vi "test_read-nmea-data2.vi"() -> ()   [LabVIEW 2019] (continued)
\t\n15:13:37.95\tF9P\t\t\n15:13:37.97\tF9P\t\t\n15:13:37.99\tF9P\t\t\n15:13:38.01\tF9P\t\t\n15:13:38.03\tF9P\t\t\n15:13:38.05\tF9P\t\t\n15:13:38.07\tF9P\t\t\n15:13:38.09\tF9P\t\t\n15:13:38.11\tF9P\t\t\n15:13:38.13\tF9P\t\t\n15:13:38.15\tF9P\t\t\n15:13:38.17\tF9P\t\t\n15:13:38.19\tF9P\t\t\n15:13:38.21\tF9P\t\t\n15:13:38.23\tF9P\t$GNRMC,061340.00,A,3723.56861,N,12656.98776,E,1.974,335.21,250720,,,A,V*0D\n\t\n15:13:38.25\tF9P\t$GNVTG,335.21,T,,M,1.974,N,3.655,K,A*2B\n\t\n15:13:38.27\tF9P\t$GNGGA,061340.00,3723.56861,N,12656.98776,E,1,12,1.09,47.7,M,18.5,M,,*79\n\t\n15:13:38.29\tF9P\t$GNGSA,A,3,12,06,19,05,17,09,04,02,,,,,2.14,1.09,1.84,1*02\n\t\n15:13:38.31\tF9P\t$GNGSA,A,3,85,70,71,84,,,,,,,,,2.14,1.09,1.84,2*00\n\t\n15:13:38.33\tF9P\t$GNGSA,A,3,36,19,11,04,09,12,,,,,,,2.14,1.09,1.84,3*02\n\t\n15:13:38.35\tF9P\t$GNGSA,A,3,14,11,33,,,,,,,,,,2.14,1.09,1.84,4*03\n\t\n15:13:38.37\tF9P\t$GPGSV,3,1,09,02,55,320,29,04,17,043,18,05,38,248,26,06,64,050,38,1*65\n\t\n15:13:38.39\tF9P\t$GPGSV,3,2,09,09,44,073,30,12,23,276,33,17,32,154,33,19,51,157,37,1*6F\n\t\n15:13:38.41\tF9P\t$GPGSV,3,3,09,25,12,306,23,1*5D\n\t\n15:13:38.43\tF9P\t$GPGSV,3,1,09,02,55,320,,04,17,043,,05,38,248,,06,64,050,25,6*68\n\t\n15:13:38.45\tF9P\t$GPGSV,3,2,09,09,44,073,27,12,23,276,30,17,32,154,23,19,51,157,,6*68\n\t\n15:13:38.47\tF9P\t$GPGSV,3,3,09,25,12,306,,6*5B\n\t\n15:13:38.49\tF9P\t$GLGSV,2,1,08,69,11,031,33,70,70,038,25,71,53,206,30,72,05,210,17,1*70\n\t\n15:13:38.51\tF9P\t$GLGSV,2,2,08,77,01,325,,84,19,123,17,85,70,070,33,86,37,330,,1*70\n\t\n15:13:38.53\tF9P\t$GLGSV,2,1,08,69,11,031,20,70,70,038,,71,53,206,23,72,05,210,,3*73\n\t\n15:13:38.55\tF9P\t$GLGSV,2,2,08,77,01,325,,84,19,123,20,85,70,070,22,86,37,330,,3*76\n\t\n15:13:38.57\tF9P\t$GAGSV,2,1,08,02,08,297,11,04,66,116,31,09,32,193,35,11,72,359,24,7*77\n\t\n15:13:38.59\tF9P\t$GAGSV,2,2,08,12,40,103,29,19,26,045,16,25,09,249,,36,26,308,14,7*71\n\t\n15:13:38.61\tF9P\t$GAGSV,2,1,08,02,08,297,,04,66,116,,09,32,193,,11,72,359,,2*70\n\t\n15:13:38.63\tF9P\t$GAGSV,2,2,08,12,40,103,,19,26,045,,25,09,249,,36,26,308,,2*7D\n\t\n15:13:38.65\tF9P\t$GBGSV,1,1,04,11,49,132,30,14,87,114,27,28,,,34,33,61,220,21,1*4E\n\t\n15:13:38.67\tF9P\t$GBGSV,1,1,03,11,49,132,34,14,87,114,,33,61,220,,3*44\n\t\n15:13:38.69\tF9P\t$GNGLL,3723.56861,N,12656.98776,E,061340.00,A,A*7F\n\t\n15:13:38.71\tF9P\t\t\n15:13:38.73\tF9P\t\t\n15:13:38.75\tF9P\t\t\n15:13:38.77\tF9P\t\t\n15:13:38.79\tF9P\t\t\n15:13:38.81\tF9P\t\t\n15:13:38.83\tF9P\t\t\n15:13:38.85\tF9P\t\t\n15:13:38.87\tF9P\t\t\n15:13:38.89\tF9P\t\t\n15:13:38.91\tF9P\t\t\n15:13:38.93\tF9P\t\t\n15:13:38.95\tF9P\t\t\n15:13:38.97\tF9P\t\t\n15:13:38.99\tF9P\t\t\n15:13:39.01\tF9P\t\t\n15:13:39.03\tF9P\t\t\n15:13:39.05\tF9P\t\t\n15:13:39.07\tF9P\t\t\n15:13:39.09\tF9P\t\t\n15:13:39.11\tF9P\t\t\n15:13:39.13\tF9P\t\t\n15:13:39.15\tF9P\t\t\n15:13:39.17\tF9P\t\t\n15:13:39.19\tF9P\t\t\n15:13:39.21\tF9P\t\t\n15:13:39.23\tF9P\t$GNRMC,061341.00,A,3723.56927,N,12656.98763,E,2.191,340.11,250720,,,A,V*0A\n\t\n15:13:39.25\tF9P\t$GNVTG,340.11,T,,M,2.191,N,4.057,K,A*29\n\t\n15:13:39.27\tF9P\t$GNGGA,061341.00,3723.56927,N,12656.98763,E,1,12,1.09,47.1,M,18.5,M,,*79\n\t\n15:13:39.29\tF9P\t$GNGSA,A,3,12,06,19,05,17,09,04,02,,,,,2.14,1.09,1.84,1*02\n\t\n15:13:39.31\tF9P\t$GNGSA,A,3,85,70,71,84,,,,,,,,,2.14,1.09,1.84,2*00\n\t\n15:13:39.33\tF9P\t$GNGSA,A,3,36,19,11,04,09,12,,,,,,,2.14,1.09,1.84,3*02\n\t\n15:13:39.35\tF9P\t$GNGSA,A,3,14,11,33,,,,,,,,,,2.14,1.09,1.84,4*03\n\t\n15:13:39.37\tF9P\t$GPGSV,3,1,09,02,55,320,32,04,17,043,19,05,38,248,25,06,64,050,31,1*64\n\t\n15:13:39.39\tF9P\t$GPGSV,3,2,09,09,44,073,36,12,23,276,37,17,32,154,36,19,51,157,41,1*69\n\t\n15:13:39.41\tF9P\t$GPGSV,3,3,09,25,12,306,23,1*5D\n\t\n15:13:39.43\tF9P\t$GPGSV,3,1,09,02,55,320,,04,17,043,,05,38,248,,06,64,050,25,6*68\n\t\n15:13:39.45\tF9P\t$GPGSV,3,2,09,09,44,073,28,12,23,276,28,17,32,154,24,19,51,157,,6*69\n\t\n15:13:39.47\tF9P\t$GPGSV,3,3,09,25,12,306,,6*5B\n\t\n15:13:39.49\tF9P\t$GLGSV,2,1,08,69,11,031,19,70,70,038,24,71,53,206,29,72,05,210,17,1*71\n\t\n15:13:39.51\tF9P\t$GLGSV,2,2,08,77,01,325,,84,19,123,17,85,70,070,29,86,37,330,,1*7B\n\t\n15:13:39.53\tF9P\t$GLGSV,2,1,08,69,11,031,20,70,70,038,,71,53,206,22,72,05,210,,3*72\n\t\n15:13:39.55\tF9P\t$GLGSV,2,2,08,77,01,325,,84,19,123,21,85,70,070,21,86,37,330,,3*74\n\t\n15:13:39.57\tF9P\t$GAGSV,2,1,08,02,08,297,09,04,66,116,26,09,32,193,28,11,72,359,25,7*75\n\t\n15:13:39.59\tF9P\t$GAGSV,2,2,08,12,40,103,30,19,26,045,16,25,09,249,,36,26,308,14,7*79\n\t\n15:13:39.61\tF9P\t$GAGSV,2,1,08,02,08,297,,04,66,116,,09,32,193,,11,72,359,,2*70\n\t\n15:13:39.63\tF9P\t$GAGSV,2,2,08,12,40,103,,19,26,045,,25,09,249,,36,26,308,,2*7D\n\t\n15:13:39.65\tF9P\t$GBGSV,1,1,04,11,49,132,31,14,87,114,32,28,,,25,33,61,220,21,1*4B\n\t\n15:13:39.67\tF9P\t$GBGSV,1,1,03,11,49,132,31,14,87,114,31,33,61,220,,3*43\n\t\n15:13:39.69\tF9P\t$GNGLL,3723.56927,N,12656.98763,E,061341.00,A,A*79\n\t\n15:13:39.71\tF9P\t\t\n15:13:39.73\tF9P\t\t\n15:13:39.75\tF9P\t\t\n15:13:39.77\tF9P\t\t\n15:13:39.79\tF9P\t\t\n15:13:39.81\tF9P\t\t\n15:13:39.83\tF9P\t\t\n15:13:39.85\tF9P\t\t\n15:13:39.87\tF9P\t\t\n15:13:39.89\tF9P\t\t\n15:13:39.91\tF9P\t\t\n15:13:39.93\tF9P\t\t\n15:13:39.95\tF9P\t\t\n15:13:39.97\tF9P\t\t\n15:13:39.99\tF9P\t\t\n15:13:40.01\tF9P\t\t\n15:13:40.03\tF9P\t\t\n15:13:40.05\tF9P\t\t\n15:13:40.07\tF9P\t\t\n15:13:40.09\tF9P\t\t\n15:13:40.11\tF9P\t\t\n15:13:40.13\tF9P\t\t\n15:13:40.15\tF9P\t\t\n15:13:40.17\tF9P\t\t\n15:13:40.19\tF9P\t\t\n15:13:40.21\tF9P\t\t\n15:13:40.23\tF9P\t$GNRMC,061342.00,A,3723.56991,N,12656.98768,E,1.862,343.66,250720,,,A,V*0A\n\t\n15:13:40.25\tF9P\t$GNVTG,343.66,T,,M,1.862,N,3.449,K,A*20\n\t\n15:13:40.27\tF9P\t$GNGGA,061342.00,3723.56991,N,12656.98768,E,1,12,1.09,46.8,M,18.5,M,,*74\n\t\n15:13:40.29\tF9P\t$GNGSA,A,3,12,06,19,05,17,09,04,02,,,,,2.14,1.09,1.84,1*02\n\t\n15:13:40.31\tF9P\t$GNGSA,A,3,85,70,71,84,,,,,,,,,2.14,1.09,1.84,2*00\n\t\n15:13:40.33\tF9P\t$GNGSA,A,3,36,19,11,04,09,12,,,,,,,2.14,1.09,1.84,3*02\n\t\n15:13:40.35\tF9P\t$GNGSA,A,3,14,11,33,,,,,,,,,,2.14,1.09,1.84,4*03\n\t\n15:13:40.37\tF9P\t$GPGSV,3,1,09,02,55,320,27,04,17,043,20,05,38,248,26,06,64,050,35,1*6D\n\t\n15:13:40.39\tF9P\t$GPGSV,3,2,09,09,44,073,38,12,23,276,32,17,32,154,31,19,51,157,37,1*64\n\t\n15:13:40.41\tF9P\t$GPGSV,3,3,09,25,12,306,20,1*5E\n\t\n15:13:40.43\tF9P\t$GPGSV,3,1,09,02,55,320,,04,17,043,,05,38,248,,06,64,050,26,6*6B\n\t\n15:13:40.45\tF9P\t$GPGSV,3,2,09,09,44,073,28,12,23,276,21,17,32,154,25,19,51,157,,6*61\n\t\n15:13:40.47\tF9P\t$GPGSV,3,3,09,25,12,306,,6*5B\n\t\n15:13:40.49\tF9P\t$GLGSV,2,1,08,69,11,031,29,70,70,038,25,71,53,206,29,72,05,210,17,1*73\n\t\n15:13:40.51\tF9P\t$GLGSV,2,2,08,77,01,325,,84,19,123,19,85,70,070,32,86,37,330,,1*7F\n\t\n15:13:40.53\tF9P\t$GLGSV,2,1,08,69,11,031,20,70,70,038,,71,53,206,20,72,05,210,,3*70\n\t\n15:13:40.55\tF9P\t$GLGSV,2,2,08,77,01,325,,84,19,123,24,85,70,070,21,86,37,330,,3*71\n\t\n15:13:40.57\tF9P\t$GAGSV,2,1,08,02,08,297,12,04,66,116,26,09,32,193,32,11,72,359,25,7*74\n\t\n15:13:40.59\tF9P\t$GAGSV,2,2,08,12,40,103,30,19,26,045,16,25,09,249,,36,26,308,12,7*7F\n\t\n15:13:40.61\tF9P\t$GAGSV,2,1,08,02,08,297,,04,66,116,,09,32,193,,11,72,359,,2*70\n\t\n15:13:40.63\tF9P\t$GAGSV,2,2,08,12,40,103,,19,26,045,,25,09,249,,36,26,308,,2*7D\n\t\n15:13:40.65\tF9P\t$GBGSV,1,1,04,11,49,132,30,14,87,114,29,28,,,30,33,61,220,22,1*47\n\t\n15:13:40.67\tF9P\t$GBGSV,1,1,03,11,49,132,27,14,87,114,32,33,61,220,,3*47\n\t\n15:13:40.69\tF9P\t$GNGLL,3723.56991,N,12656.98768,E,061342.00,A,A*7C\n\t\n15:13:40.71\tF9P\t\t\n15:13:40.73\tF9P\t\t\n15:13:40.75\tF9P\t\t\n15:13:40.77\tF9P\t\t\n15:13:40.79\tF9P\t\t\n15:13:40.81\tF9P\t\t\n15:13:40.83\tF9P\t\t\n15:13:40.85\tF9P\t\t\n15:13:40.87\tF9P\t\t\n15:13:40.89\tF9P\t\t\n15:13:40.91\tF9P\t\t\n15:13:40.93\tF9P\t\t\n15:13:40.95\tF9P\t\t\n15:13:40.97\tF9P\t\t\n15:13:40.99\tF9P\t\t\n15:13:41.01\tF9P\t\t\n15:13:41.03\tF9P\t\t\n15:13:41.05\tF9P\t\t\n15:13:41.07\tF9P\t\t\n15:13:41.09\tF9P\t\t\n15:13:41.11\tF9P\t\t\n15:13:41.13\tF9P\t\t\n15:13:41.15\tF9P\t\t\n15:13:41.17\tF9P\t\t\n15:13:41.19\tF9P\t\t\n15:13:41.21\tF9P\t\t\n15:13:41.23\tF9P\t$GNRMC,061343.00,A,3723.57038,N,12656.98785,E,1.526,349.41,250720,,,A,V*01\n\t\n15:13:41.25\tF9P\t$GNVTG,349.41,T,,M,1.526,N,2.827,K,A*27\n\t\n15:13:41.27\tF9P\t$GNGGA,061343.00,3723.57038,N,12656.98785,E,1,12,1.09,46.8,M,18.5,M,,*7D\n\t\n15:13:41.29\tF9P\t$GNGSA,A,3,12,06,19,05,17,09,04,02,,,,,2.14,1.09,1.84,1*02\n\t\n15:13:41.31\tF9P\t$GNGSA,A,3,85,70,71,84,,,,,,,,,2.14,1.09,1.84,2*00\n\t\n15:13:41.33\tF9P\t$GNGSA,A,3,36,19,11,04,09,12,,,,,,,2.14,1.09,1.84,3*02\n\t\n15:13:41.35\tF9P\t$GNGSA,A,3,14,11,33,,,,,,,,,,2.14,1.09,1.84,4*03\n\t\n15:13:41.37\tF9P\t$GPGSV,3,1,09,02,55,320,32,04,17,043,20,05,38,248,26,06,64,050,26,1*6B\n\t\n15:13:41.39\tF9P\t$GPGSV,3,2,09,09,44,073,35,12,23,276,34,17,32,154,33,19,51,157,40,1*6D\n\t\n15:13:41.41\tF9P\t$GPGSV,3,3,09,25,12,306,19,1*54\n\t\n15:13:41.43\tF9P\t$GPGSV,3,1,09,02,55,320,,04,17,043,,05,38,248,,06,64,050,25,6*68\n\t\n15:13:41.45\tF9P\t$GPGSV,3,2,09,09,44,073,27,12,23,276,22,17,32,154,24,19,51,157,,6*6C\n\t\n15:13:41.47\tF9P\t$GPGSV,3,3,09,25,12,306,,6*5B\n\t\n15:13:41.49\tF9P\t$GLGSV,2,1,08,69,11,031,39,70,70,038,24,71,53,206,30,72,05,210,18,1*74\n\t\n15:13:41.51\tF9P\t$GLGSV,2,2,08,77,01,325,,84,19,123,21,85,70,070,30,86,37,330,,1*76\n\t\n15:13:41.53\tF9P\t$GLGSV,2,1,08,69,11,031,19,70,70,038,,71,53,206,21,72,05,210,,3*7B\n\t\n15:13:41.55\tF9P\t$GLGSV,2,2,08,77,01,325,,84,19,123,25,85,70,070,21,86,37,330,,3*70\n\t\n15:13:41.57\tF9P\t$GAGSV,2,1,08,02,08,297,09,04,66,116,32,09,32,193,33,11,72,359,24,7*7B\n\t\n15:13:41.59\tF9P\t$GAGSV,2,2,08,12,40,103,30,19,26,045,16,25,09,249,,36,26,308,11,7*7C\n\t\n15:13:41.61\tF9P\t$GAGSV,2,1,08,02,08,297,,04,66,116,,09,32,193,,11,72,359,,2*70\n\t\n15:13:41.63\tF9P\t$GAGSV,2,2,08,12,40,103,,19,26,045,,25,09,249,,36,26,308,,2*7D\n\t\n15:13:41.65\tF9P\t$GBGSV,1,1,04,11,49,132,30,14,87,114,28,28,,,30,33,61,220,25,1*41\n\t\n15:13:41.67\tF9P\t$GBGSV,1,1,03,11,49,132,32,14,87,114,31,33,61,220,,3*40\n\t\n15:13:41.69\tF9P\t$GNGLL,3723.57038,N,12656.98785,E,061343.00,A,A*75\n\t\n15:13:41.71\tF9P\t\t\n15:13:41.73\tF9P\t\t\n15:13:41.75\tF9P\t\t\n15:13:41.77\tF9P\t\t\n15:13:41.79\tF9P\t\t\n15:13:41.81\tF9P\t\t\n15:13:41.83\tF9P\t\t\n15:13:41.85\tF9P\t\t\n15:13:41.87\tF9P\t\t\n15:13:41.89\tF9P\t\t\n15:13:41.91\tF9P\t\t\n15:13:41.93\tF9P\t\t\n15:13:41.95\tF9P\t\t\n15:13:41.97\tF9P\t\t\n15:13:41.99\tF9P\t\t\n15:13:42.01\tF9P\t\t\n15:13:42.03\tF9P\t\t\n15:13:42.05\tF9P\t\t\n15:13:42.07\tF9P\t\t\n15:13:42.09\tF9P\t\t\n15:13:42.11\tF9P\t\t\n15:13:42.13\tF9P\t\t\n15:13:42.15\tF9P\t\t\n15:13:42.17\tF9P\t\t\n15:13:42.19\tF9P\t\t\n15:13:42.21\tF9P\t\t\n15:13:42.23\tF9P\t$GNRMC,061344.00,A,3723.57068,N,12656.98790,E,1.413,345.66,250720,,,A,V*09\n\t\n15:13:42.25\tF9P\t$GNVTG,345.66,T,,M,1.413,N,2.616,K,A*25\n\t\n15:13:42.27\tF9P\t$GNGGA,061344.00,3723.57068,N,12656.98790,E,1,12,0.95,47.4,M,18.5,M,,*72\n\t\n15:13:42.29\tF9P\t$GNGSA,A,3,12,06,19,05,17,09,04,02,,,,,1.88,0.95,1.62,1*08\n\t\n15:13:42.31\tF9P\t$GNGSA,A,3,85,70,71,84,,,,,,,,,1.88,0.95,1.62,2*0A\n\t\n15:13:42.33\tF9P\t$GNGSA,A,3,36,19,11,04,09,12,,,,,,,1.88,0.95,1.62,3*08\n\t\n15:13:42.35\tF9P\t$GNGSA,A,3,14,11,33,,,,,,,,,,1.88,0.95,1.62,4*09\n\t\n15:13:42.37\tF9P\t$GPGSV,3,1,09,02,55,320,30,04,17,043,21,05,38,248,30,06,64,050,31,1*69\n\t\n15:13:42.39\tF9P\t$GPGSV,3,2,09,09,44,073,27,12,23,276,40,17,32,154,33,19,51,157,36,1*6C\n\t\n15:13:42.41\tF9P\t$GPGSV,3,3,09,25,12,306,19,1*54\n\t\n15:13:42.43\tF9P\t$GPGSV,3,1,09,02,55,320,,04,17,043,,05,38,248,19,06,64,050,26,6*63\n\t\n15:13:42.45\tF9P\t$GPGSV,3,2,09,09,44,073,25,12,23,276,26,17,32,154,25,19,51,157,,6*6B\n\t\n15:13:42.47\tF9P\t$GPGSV,3,3,09,25,12,306,,6*5B\n\t\n15:13:42.49\tF9P\t$GLGSV,2,1,08,69,11,031,37,70,70,038,25,71,53,206,24,72,05,210,18,1*7E\n\t\n15:13:42.51\tF9P\t$GLGSV,2,2,08,77,01,325,,84,19,123,20,85,70,070,34,86,37,330,,1*73\n\t\n15:13:42.53\tF9P\t$GLGSV,2,1,08,69,11,031,22,70,70,038,,71,53,206,21,72,05,210,,3*73\n\t\n15:13:42.55\tF9P\t$GLGSV,2,2,08,77,01,325,,84,19,123,30,85,70,070,22,86,37,330,,3*77\n\t\n15:13:42.57\tF9P\t$GAGSV,2,1,08,02,08,297,11,04,66,116,31,09,32,193,32,11,72,359,24,7*70\n\t\n15:13:42.59\tF9P\t$GAGSV,2,2,08,12,40,103,31,19,26,045,15,25,09,249,,36,26,308,10,7*7F\n\t\n15:13:42.61\tF9P\t$GAGSV,2,1,08,02,08,297,,04,66,116,,09,32,193,,11,72,359,,2*70\n\t\n15:13:42.63\tF9P\t$GAGSV,2,2,08,12,40,103,,19,26,045,,25,09,249,,36,26,308,,2*7D\n\t\n15:13:42.65\tF9P\t$GBGSV,1,1,04,11,49,132,33,14,87,114,28,28,,,30,33,61,220,24,1*43\n\t\n15:13:42.67\tF9P\t$GBGSV,1,1,03,11,49,132,26,14,87,114,28,33,61,220,,3*4D\n\t\n15:13:42.69\tF9P\t$GNGLL,3723.57068,N,12656.98790,E,061344.00,A,A*73\n\t\n15:13:42.71\tF9P\t\t\n15:13:42.73\tF9P\t\t\n15:13:42.75\tF9P\t\t\n15:13:42.77\tF9P\t\t\n15:13:42.79\tF9P\t\t\n15:13:42.81\tF9P\t\t\n15:13:42.83\tF9P\t\t\n15:13:42.85\tF9P\t\t\n15:13:42.87\tF9P\t\t\n15:13:42.89\tF9P\t\t\n15:13:42.91\tF9P\t\t\n15:13:42.93\tF9P\t\t\n15:13:42.95\tF9P\t\t\n15:13:42.97\tF9P\t\t\n15:13:42.99\tF9P\t\t\n15:13:43.01\tF9P\t\t\n15:13:43.03\tF9P\t\t\n15:13:43.05\tF9P\t\t\n15:13:43.07\tF9P\t\t\n15:13:43.09\tF9P\t\t\n15:13:43.11\tF9P\t\t\n15:13:43.13\tF9P\t\t\n15:13:43.15\tF9P\t\t\n15:13:43.17\tF9P\t\t\n15:13:43.19\tF9P\t\t\n15:13:43.21\tF9P\t\t\n15:13:43.23\tF9P\t$GNRMC,061345.00,A,3723.57138,N,12656.98801,E,2.029,352.53,250720,,,A,V*05\n\t\n15:13:43.25\tF9P\t$GNVTG,352.53,T,,M,2.029,N,3.758,K,A*21\n\t\n15:13:43.27\tF9P\t$GNGGA,061345.00,3723.57138,N,12656.98801,E,1,12,1.09,46.9,M,18.5,M,,*78\n\t\n15:13:43.29\tF9P\t$GNGSA,A,3,12,06,19,05,17,09,04,02,,,,,2.14,1.09,1.84,1*02\n\t\n15:13:43.31\tF9P\t$GNGSA,A,3,85,70,71,84,,,,,,,,,2.14,1.09,1.84,2*00\n\t\n15:13:43.33\tF9P\t$GNGSA,A,3,36,19,11,04,09,12,,,,,,,2.14,1.09,1.84,3*02\n\t\n15:13:43.35\tF9P\t$GNGSA,A,3,14,11,33,,,,,,,,,,2.14,1.09,1.84,4*03\n\t\n15:13:43.37\tF9P\t$GPGSV,3,1,09,02,55,320,30,04,17,043,22,05,38,248,25,06,64,050,30,1*6F\n\t\n15:13:43.39\tF9P\t$GPGSV,3,2,09,09,44,073,34,12,23,276,29,17,32,154,39,19,51,157,36,1*6B\n\t\n15:13:43.41\tF9P\t$GPGSV,3,3,09,25,12,306,20,1*5E\n\t\n15:13:43.43\tF9P\t$GPGSV,3,1,09,02,55,320,,04,17,043,,05,38,248,19,06,64,050,25,6*60\n\t\n15:13:43.45\tF9P\t$GPGSV,3,2,09,09,44,073,31,12,23,276,25,17,32,154,23,19,51,157,,6*6B\n\t\n15:13:43.47\tF9P\t$GPGSV,3,3,09,25,12,306,,6*5B\n\t\n15:13:43.49\tF9P\t$GLGSV,2,1,08,69,11,031,40,70,70,038,24,71,53,206,30,72,05,210,18,1*7A\n\t\n15:13:43.51\tF9P\t$GLGSV,2,2,08,77,01,325,,84,19,123,21,85,70,070,28,86,37,330,,1*7F\n\t\n15:13:43.53\tF9P\t$GLGSV,2,1,08,69,11,031,23,70,70,038,,71,53,206,19,72,05,210,,3*79\n\t\n15:13:43.55\tF9P\t$GLGSV,2,2,08,77,01,325,,84,19,123,26,85,70,070,23,86,37,330,,3*71\n\t\n15:13:43.57\tF9P\t$GAGSV,2,1,08,02,08,297,09,04,66,116,30,09,32,193,25,11,72,359,26,7*7C\n\t\n15:13:43.59\tF9P\t$GAGSV,2,2,08,12,40,103,37,19,26,045,16,25,09,249,,36,26,308,10,7*7A\n\t\n15:13:43.61\tF9P\t$GAGSV,2,1,08,02,08,297,,04,66,116,,09,32,193,,11,72,359,,2*70\n\t\n15:13:43.63\tF9P\t$GAGSV,2,2,08,12,40,103,,19,26,045,,25,09,249,,36,26,308,,2*7D\n\t\n15:13:43.65\tF9P\t$GBGSV,1,1,04,11,49,132,36,14,87,114,27,28,,,32,33,61,220,26,1*49\n\t\n15:13:43.67\tF9P\t$GBGSV,1,1,03,11,49,132,,14,87,114,27,33,61,220,,3*46\n\t\n15:13:43.69\tF9P\t$GNGLL,3723.57138,N,12656.98801,E,061345.00,A,A*71\n\t\n15:13:43.71\tF9P\t\t\n15:13:43.73\tF9P\t\t\n15:13:43.75\tF9P\t\t\n15:13:43.77\tF9P\t\t\n15:13:43.79\tF9P\t\t\n15:13:43.81\tF9P\t\t\n15:13:43.83\tF9P\t\t\n15:13:43.85\tF9P\t\t\n15:13:43.87\tF9P\t\t\n15:13:43.89\tF9P\t\t\n15:13:43.91\tF9P\t\t\n15:13:43.93\tF9P\t\t\n15:13:43.95\tF9P\t\t\n15:13:43.97\tF9P\t\t\n15:13:43.99\tF9P\t\t\n15:13:44.01\tF9P\t\t\n15:13:44.03\tF9P\t\t\n15:13:44.05\tF9P\t\t\n15:13:44.07\tF9P\t\t\n15:13:44.09\tF9P\t\t\n15:13:44.11\tF9P\t\t\n15:13:44.13\tF9P\t\t\n15:13:44.15\tF9P\t\t\n15:13:44.17\tF9P\t\t\n15:13:44.19\tF9P\t\t\n15:13:44.21\tF9P\t\t\n15:13:44.23\tF9P\t$GNRMC,061346.00,A,3723.57187,N,12656.98793,E,1.946,345.99,250720,,,A,V*05\n\t\n15:13:44.25\tF9P\t$GNVTG,345.99,T,,M,1.946,N,3.605,K,A*2B\n\t\n15:13:44.27\tF9P\t$GNGGA,061346.00,3723.57187,N,12656.98793,E,1,12,0.82,47.1,M,18.5,M,,*70\n\t\n15:13:44.29\tF9P\t$GNGSA,A,3,12,06,19,05,17,09,04,02,,,,,1.52,0.82,1.28,1*07\n\t\n15:13:44.31\tF9P\t$GNGSA,A,3,85,70,71,84,,,,,,,,,1.52,0.82,1.28,2*05\n\t\n15:13:44.33\tF9P\t$GNGSA,A,3,36,19,11,04,09,12,,,,,,,1.52,0.82,1.28,3*07\n\t\n15:13:44.35\tF9P\t$GNGSA,A,3,14,11,33,,,,,,,,,,1.52,0.82,1.28,4*06\n\t\n15:13:44.37\tF9P\t$GPGSV,3,1,09,02,55,320,33,04,17,043,22,05,38,248,31,06,64,050,29,1*61\n\t\n15:13:44.39\tF9P\t$GPGSV,3,2,09,09,44,073,32,12,23,276,40,17,32,154,33,19,51,157,34,1*6A\n\t\n15:13:44.41\tF9P\t$GPGSV,3,3,09,25,12,306,19,1*54\n\t\n15:13:44.43\tF9P\t$GPGSV,3,1,09,02,55,320,,04,17,043,20,05,38,248,18,06,64,050,24,6*62\n\t\n15:13:44.45\tF9P\t$GPGSV,3,2,09,09,44,073,24,12,23,276,24,17,32,154,23,19,51,157,,6*6E\n\t\n15:13:44.47\tF9P\t$GPGSV,3,3,09,25,12,306,,6*5B\n\t\n15:13:44.49\tF9P\t$GLGSV,2,1,08,69,11,031,38,70,70,038,24,71,53,206,24,72,05,210,18,1*70\n\t\n15:13:44.51\tF9P\t$GLGSV,2,2,08,77,01,325,,84,19,123,22,85,70,070,32,86,37,330,,1*77\n\t\n15:13:44.53\tF9P\t$GLGSV,2,1,08,69,11,031,28,70,70,038,,71,53,206,18,72,05,210,,3*73\n\t\n15:13:44.55\tF9P\t$GLGSV,2,2,08,77,01,325,,84,19,123,25,85,70,070,23,86,37,330,,3*72\n\t\n15:13:44.57\tF9P\t$GAGSV,2,1,08,02,08,297,08,04,66,116,30,09,32,193,26,11,72,359,26,7*7E\n\t\n15:13:44.59\tF9P\t$GAGSV,2,2,08,12,40,103,25,19,26,045,15,25,09,249,,36,26,308,11,7*7B\n\t\n15:13:44.61\tF9P\t$GAGSV,2,1,08,02,08,297,,04,66,116,,09,32,193,,11,72,359,,2*70\n\t\n15:13:44.63\tF9P\t$GAGSV,2,2,08,12,40,103,,19,26,045,,25,09,249,,36,26,308,,2*7D\n\t\n15:13:44.65\tF9P\t$GBGSV,1,1,04,11,49,132,27,14,87,114,28,28,,,35,33,61,220,26,1*41\n\t\n15:13:44.67\tF9P\t$GBGSV,1,1,03,11,49,132,,14,87,114,32,33,61,220,,3*42\n\t\n15:13:44.69\tF9P\t$GNGLL,3723.57187,N,12656.98793,E,061346.00,A,A*72\n\t\n15:13:44.71\tF9P\t\t\n15:13:44.73\tF9P\t\t\n15:13:44.75\tF9P\t\t\n15:13:44.77\tF9P\t\t\n15:13:44.79\tF9P\t\t\n15:13:44.81\tF9P\t\t\n15:13:44.83\tF9P\t\t\n15:13:44.85\tF9P\t\t\n15:13:44.87\tF9P\t\t\n15:13:44.89\tF9P\t\t\n15:13:44.91\tF9P\t\t\n15:13:44.93\tF9P\t\t\n15:13:44.95\tF9P\t\t\n15:13:44.97\tF9P\t\t\n15:13:44.99\tF9P\t\t\n15:13:45.01\tF9P\t\t\n15:13:45.03\tF9P\t\t\n15:13:45.05\tF9P\t\t\n15:13:45.07\tF9P\t\t\n15:13:45.09\tF9P\t\t\n15:13:45.11\tF9P\t\t\n15:13:45.13\tF9P\t\t\n15:13:45.15\tF9P\t\t\n15:13:45.17\tF9P\t\t\n15:13:45.19\tF9P\t\t\n15:13:45.21\tF9P\t\t\n15:13:45.23\tF9P\t$GNRMC,061347.00,A,3723.57229,N,12656.98820,E,1.828,350.47,250720,,,A,V*0A\n\t\n15:13:45.25\tF9P\t$GNVTG,350.47,T,,M,1.828,N,3.385,K,A*28\n\t\n15:13:45.27\tF9P\t$GNGGA,061347.00,3723.57229,N,12656.98820,E,1,12,0.67,47.4,M,18.5,M,,*7F\n\t\n15:13:45.29\tF9P\t$GNGSA,A,3,12,06,19,05,17,09,04,02,,,,,1.24,0.67,1.04,1*03\n\t\n15:13:45.31\tF9P\t$GNGSA,A,3,85,70,71,84,,,,,,,,,1.24,0.67,1.04,2*01\n\t\n15:13:45.33\tF9P\t$GNGSA,A,3,36,19,11,04,09,12,,,,,,,1.24,0.67,1.04,3*03\n\t\n15:13:45.35\tF9P\t$GNGSA,A,3,14,11,33,,,,,,,,,,1.24,0.67,1.04,4*02\n\t\n15:13:45.37\tF9P\t$GPGSV,3,1,09,02,55,320,29,04,17,043,23,05,38,248,27,06,64,050,35,1*61\n\t\n15:13:45.39\tF9P\t$GPGSV,3,2,09,09,44,073,30,12,23,276,40,17,32,154,36,19,51,157,34,1*6D\n\t\n15:13:45.41\tF9P\t$GPGSV,3,3,09,25,12,306,18,1*55\n\t\n15:13:45.43\tF9P\t$GPGSV,3,1,09,02,55,320,,04,17,043,18,05,38,248,18,06,64,050,24,6*69\n\t\n15:13:45.45\tF9P\t$GPGSV,3,2,09,09,44,073,24,12,23,276,23,17,32,154,22,19,51,157,,6*68\n\t\n15:13:45.47\tF9P\t$GPGSV,3,3,09,25,12,306,,6*5B\n\t\n15:13:45.49\tF9P\t$GLGSV,2,1,08,69,11,031,38,70,70,038,25,71,53,206,25,72,05,210,17,1*7F\n\t\n15:13:45.51\tF9P\t$GLGSV,2,2,08,77,01,325,,84,19,123,23,85,70,070,35,86,37,330,,1*71\n\t\n15:13:45.53\tF9P\t$GLGSV,2,1,08,69,11,031,26,70,70,038,,71,53,206,17,72,05,210,,3*72\n\t\n15:13:45.55\tF9P\t$GLGSV,2,2,08,77,01,325,,84,19,123,24,85,70,070,23,86,37,330,,3*73\n\t\n15:13:45.57\tF9P\t$GAGSV,2,1,08,02,08,297,11,04,66,116,25,09,32,193,26,11,72,359,26,7*72\n\t\n15:13:45.59\tF9P\t$GAGSV,2,2,08,12,40,103,34,19,26,045,16,25,09,249,21,36,26,308,13,7*79\n\t\n15:13:45.61\tF9P\t$GAGSV,2,1,08,02,08,297,,04,66,116,,09,32,193,,
